vi "Login UI.vi"() -> ()   [LabVIEW 2016]
doc: "用户登录界面"
uses:
  Ctrls/Wizard_OK Button.ctl
  Ctrls/Wizard_Cancel Button.ctl
panel:
  in  "Cancel":T1
  in  "OK":T2
  in  "password":string caption="密  码"
  in  "name":string caption="用户名"
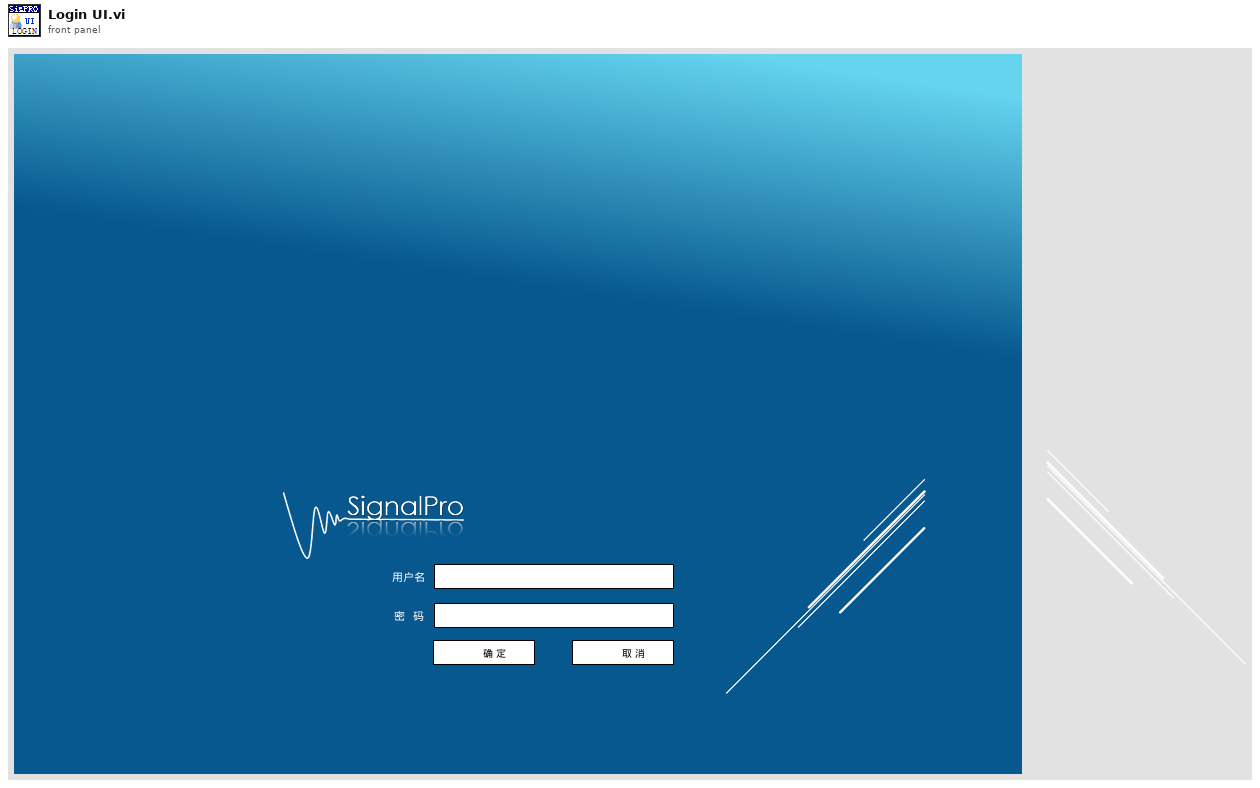
[diagram p1: front panel]
types:
  T1 = typedef "Wizard_Cancel Button.ctl" = bool
  T2 = typedef "Wizard_OK Button.ctl" = bool
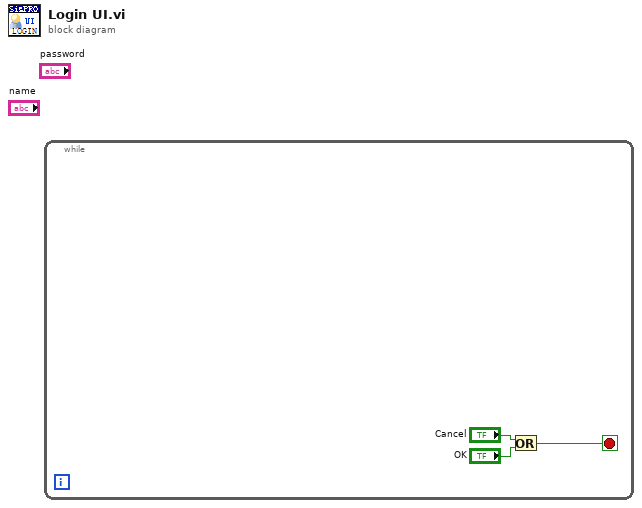
[diagram p0: block diagram]
diagram:
  n1 = while {
    stop <- w1 stop-if-true
    n2 = Or(x="Cancel", y="OK") -> (x .or. y?=w1:T1)
  }
